vi "Localize VIs.vi"(6 "Prompt user for new dictionary languages? (T)":bool=TRUE, 8 "error in (no error)":errorcluster, 10 "Dictionary Path":path, 11 "VIs in":refnum<vi>[](array[refnum])) -> (0 "error out":errorcluster)   [LabVIEW 2017, in "JKI Simple Localization.lvlib"]
uses:
  JKI Simple Localization.lvlib
  Definitions/Dictionary--Cluster.ctl
  Definitions/Private/FontCluster.ctl
  Definitions/Private/Phrase Dictionary.ctl
panel:
  out "Text Written (for debug)":string
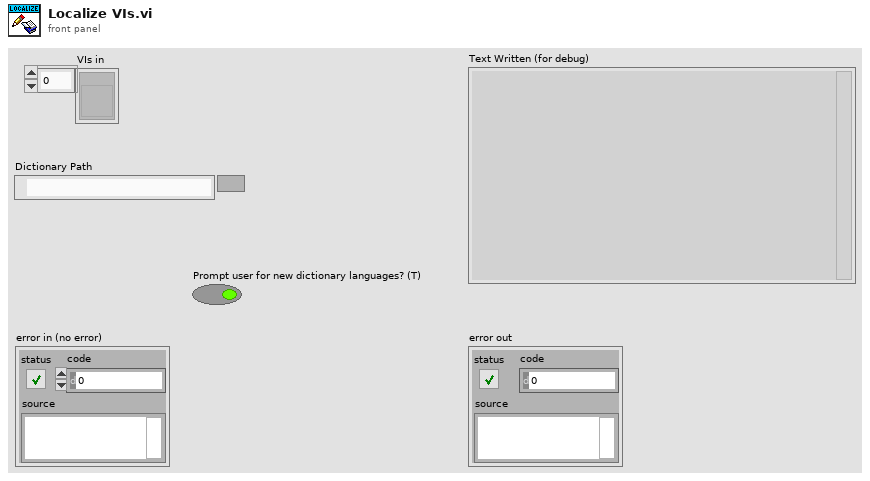
[diagram p1: front panel]
types:
  T1 = typedef "JKI Simple Localization.lvlib/Dictionary--Cluster.ctl" = cluster{"Languages":string[], "Fonts":T2[], "Phrase Dictionary":T3[]}
  T2 = typedef "JKI Simple Localization.lvlib/FontCluster.ctl" = cluster{"Language":string, "Name":string, "Color":u32}
  T3 = typedef "JKI Simple Localization.lvlib/Phrase Dictionary.ctl" = cluster{"Key":string, "Phrases":string[]}
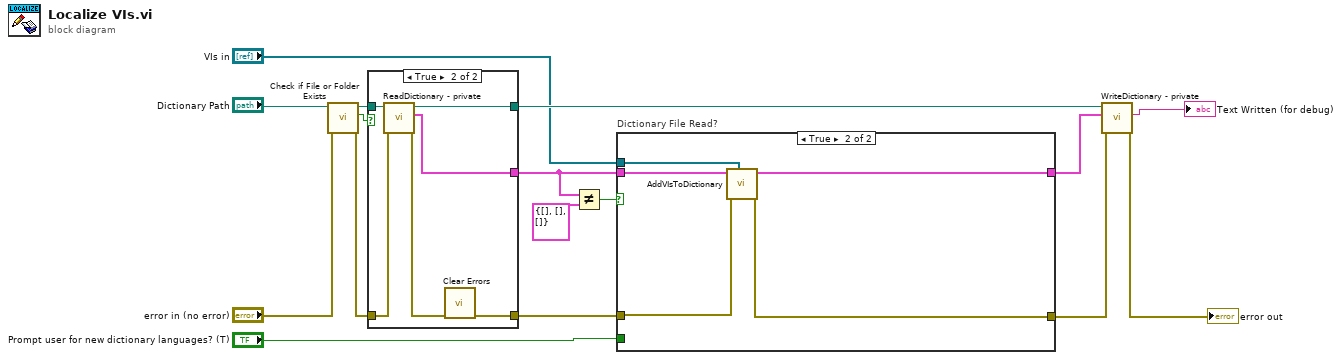
[diagram p0: block diagram]
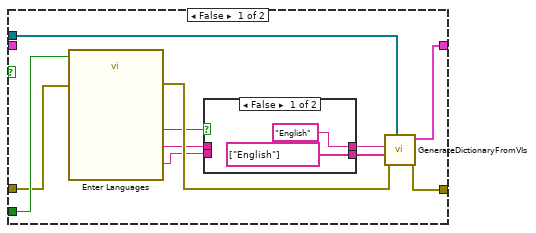
[diagram p3: hidden frame]
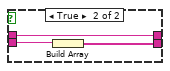
[diagram p4: hidden frame]
diagram:
  n1 = call <vilib>:"Check if File or Folder Exists.vi"("error in (no error)"="error in (no error)", "path"="Dictionary Path") -> ("error out"=w12:errorcluster, "file or folder exists?"=w11:bool, "dup path"=w13:path)  [unwired: 7 in]
  n2 = case shown="True" w11 {
    tunnel: [w18 w24] -> w15
    tunnel: w13 -> [w18 w23]
    tunnel: w12 -> [w17 w22]
    tunnel: [w17 w19] -> w9
    tunnel: [_ w20] -> w5
    frame False {
    }
    frame True {
      n3 = call "ReadDictionary - private.vi"("error in (no error)"=w22, "Dictionary File Path"=w23) -> ("error out"=w21:errorcluster, "Dictionary"=w20:T1, "Dictionary File Path out"=w24:path)  [unwired: 6 in, 1 out]
      n4 = call <vilib>:"Clear Errors.vi"("error in (no error)"=w21) -> ("error out"=w19:errorcluster)  [unwired: 5 in, 1 out]
    }
  }
  n5 = Not Equal?(x=w5, y=T1 {"Languages"=[], "Fonts"=[], "Phrase Dictionary"=[]} ("Dictionary")) -> (x != y?=w4:bool)
  n6 = case "Dictionary File Read?" shown="True" w4 {
    tunnel: w5 -> [_ w45]
    tunnel: "VIs in" -> [w35 w44]
    tunnel: w9 -> [w31 w43]
    tunnel: [w33 w42] -> w7
    tunnel: [w34 w41] -> w2
    tunnel: "Prompt user for new dictionary languages? (T)" -> [w32 _]
    frame False {
      n7 = call "Enter Languages"("Enable"=w32, "error in (no error)"=w31) -> ("Additional Language"=w27:string, "Current Language"=w28:string, "OK"=w29:bool, "error out"=w30:errorcluster)  [unwired: 14 in]
      n8 = case shown="False" w29 {
        tunnel: w28 -> [_ w39]
        tunnel: w27 -> [_ w40]
        tunnel: ["English" ("Current Language") w39] -> w26
        tunnel: [string[] ["English"] w38] -> w25
        frame False {
        }
        frame True {
          n9 = Build Array(w40) -> (w38:string[])
        }
      }
      n10 = call "GenerateDictionaryFromVIs.vi"("VIs in"=w35, "error in (no error)"=w30, "Additional Languages [English]"=w25, "Current VI Language (English)"=w26) -> ("error out"=w33:errorcluster, "Localization"=w34:T1)  [unwired: 6 in]
    }
    frame True {
      # "Add the VI text to the existing dictionary"
      n11 = call "AddVIsToDictionary.vi"("VIs in"=w44, "error in (no error)"=w43, "Dictionary from File"=w45) -> ("error out"=w42:errorcluster, "Merged Dictionary"=w41:T1)  [unwired: 7 in]
    }
  }
  n12 = call "WriteDictionary - private.vi"("error in (no error)"=w7, "Localization"=w2, "Dictionary Path"=w15) -> ("error out"=→"error out":errorcluster, "JSON String"=→"Text Written (for debug)":string)  [unwired: 6 in, 1 out]
